vi "serial-read-subVi-safe-copy.vi"() -> ()   [LabVIEW 2021]
uses:
  <vilib>/Instr/_visa.llb/VISA Configure Serial Port (Instr).vi
  SCD41.ctl
  STC31.ctl
  SHT41.ctl
  all-sensor-data.ctl
  SDP810.ctl
panel:
  out "RHT4":T1 {"Humidity (%)" format="%.2f"; "Temp (degC)" format="%.2f"}
  out "RHT3":T1 {"Humidity (%)" format="%.2f"; "Temp (degC)" format="%.2f"}
  out "RHT6":T1 {"Humidity (%)" format="%.2f"; "Temp (degC)" format="%.2f"}
  out "RHT5":T1 {"Humidity (%)" format="%.2f"; "Temp (degC)" format="%.2f"}
  out "CD6":T2 {"CO2 (ppm)" format="%.2f"}
  out "CD5":T2 {"CO2 (ppm)" format="%.2f"}
  out "CD4":T2 {"CO2 (ppm)" format="%.2f"}
  out "CD3":T2 {"CO2 (ppm)" format="%.2f"}
  out "CD2":T3 {"Humidity (%)" format="%.2f"; "Temp (degC)" format="%.2f"; "CO2 (ppm)" format="%.2f"}
  out "CD1":T3 {"Humidity (%)" format="%.2f"; "Temp (degC)" format="%.2f"; "CO2 (ppm)" format="%.2f"}
  out "all-sensor-data":T4 {"dP3"."Temp (degC)" format="%.2f"; "dP3"."dP (mBar)" format="%.2f"; "dP2"."Temp (degC)" format="%.2f"; "dP2"."dP (mBar)" format="%.2f"; "dP1"."Temp (degC)" format="%.2f"; "dP1"."dP (mBar)" format="%.2f"; "CD4"."CO2 (ppm)" format="%.2f"; "CD3"."CO2 (ppm)" format="%.2f"; "RHT4"."Humidity (%)" format="%.2f"; "RHT4"."Temp (degC)" format="%.2f"; "RHT5"."Humidity (%)" format="%.2f"; "RHT5"."Temp (degC)" format="%.2f"; "CD2"."Humidity (%)" format="%.2f"; "CD2"."Temp (degC)" format="%.2f"; "CD2"."CO2 (ppm)" format="%.2f"; "RHT3"."Humidity (%)" format="%.2f"; "RHT3"."Temp (degC)" format="%.2f"; "CD6"."CO2 (ppm)" format="%.2f"; "RHT6"."Humidity (%)" format="%.2f"; "RHT6"."Temp (degC)" format="%.2f"; "CD5"."CO2 (ppm)" format="%.2f"; "CD1"."Humidity (%)" format="%.2f"; "CD1"."Temp (degC)" format="%.2f"; "CD1"."CO2 (ppm)" format="%.2f"}
  in  "state":string
  out "Num Samples":i32
  out "error out":errorcluster
  out "data string array":string[](array[string])
  out "read buffer":string
  out "Bytes Returned":u32
  in  "VISA resource name":refnum<visa-resource-name>="COM22"
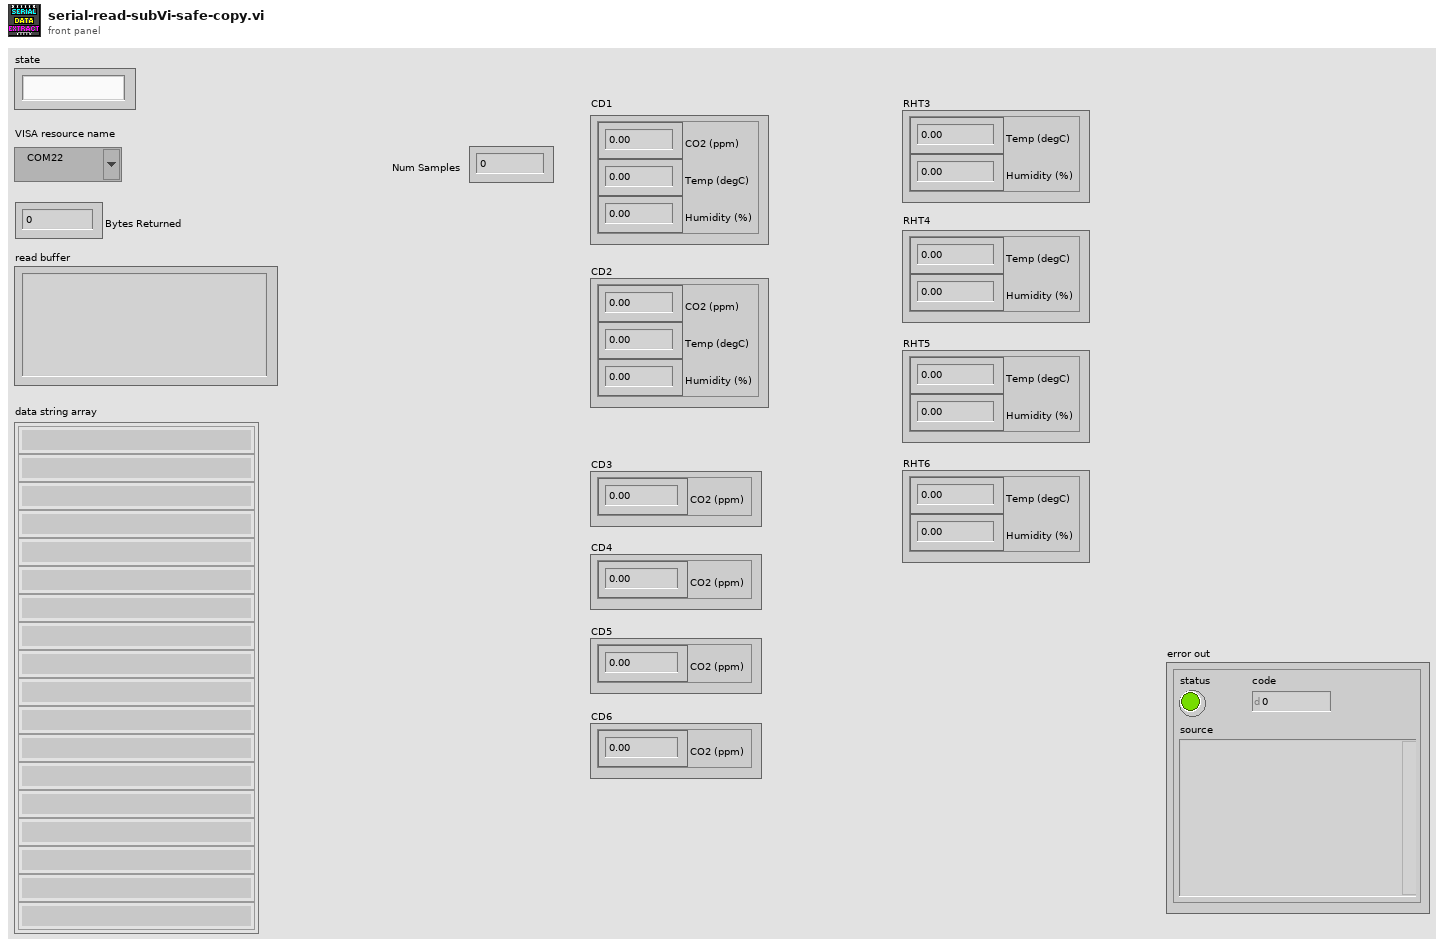
[diagram p1: front panel]
types:
  T1 = typedef "SHT41.ctl" = cluster{"Temp (degC)":dbl, "Humidity (%)":dbl}
  T2 = typedef "STC31.ctl" = cluster{"CO2 (ppm)":dbl}
  T3 = typedef "SCD41.ctl" = cluster{"CO2 (ppm)":dbl, "Temp (degC)":dbl, "Humidity (%)":dbl}
  T4 = typedef "all-sensor-data.ctl" = cluster{"CD1":T3, "CD2":T3, "CD3":T2, "CD4":T2, "CD5":T2, "CD6":T2, "RHT3":T1, "RHT4":T1, "RHT5":T1, "RHT6":T1, "dP1":T5, "dP2":T5, "dP3":T5}
  T5 = typedef "SDP810.ctl" = cluster{"dP (mBar)":dbl, "Temp (degC)":dbl}
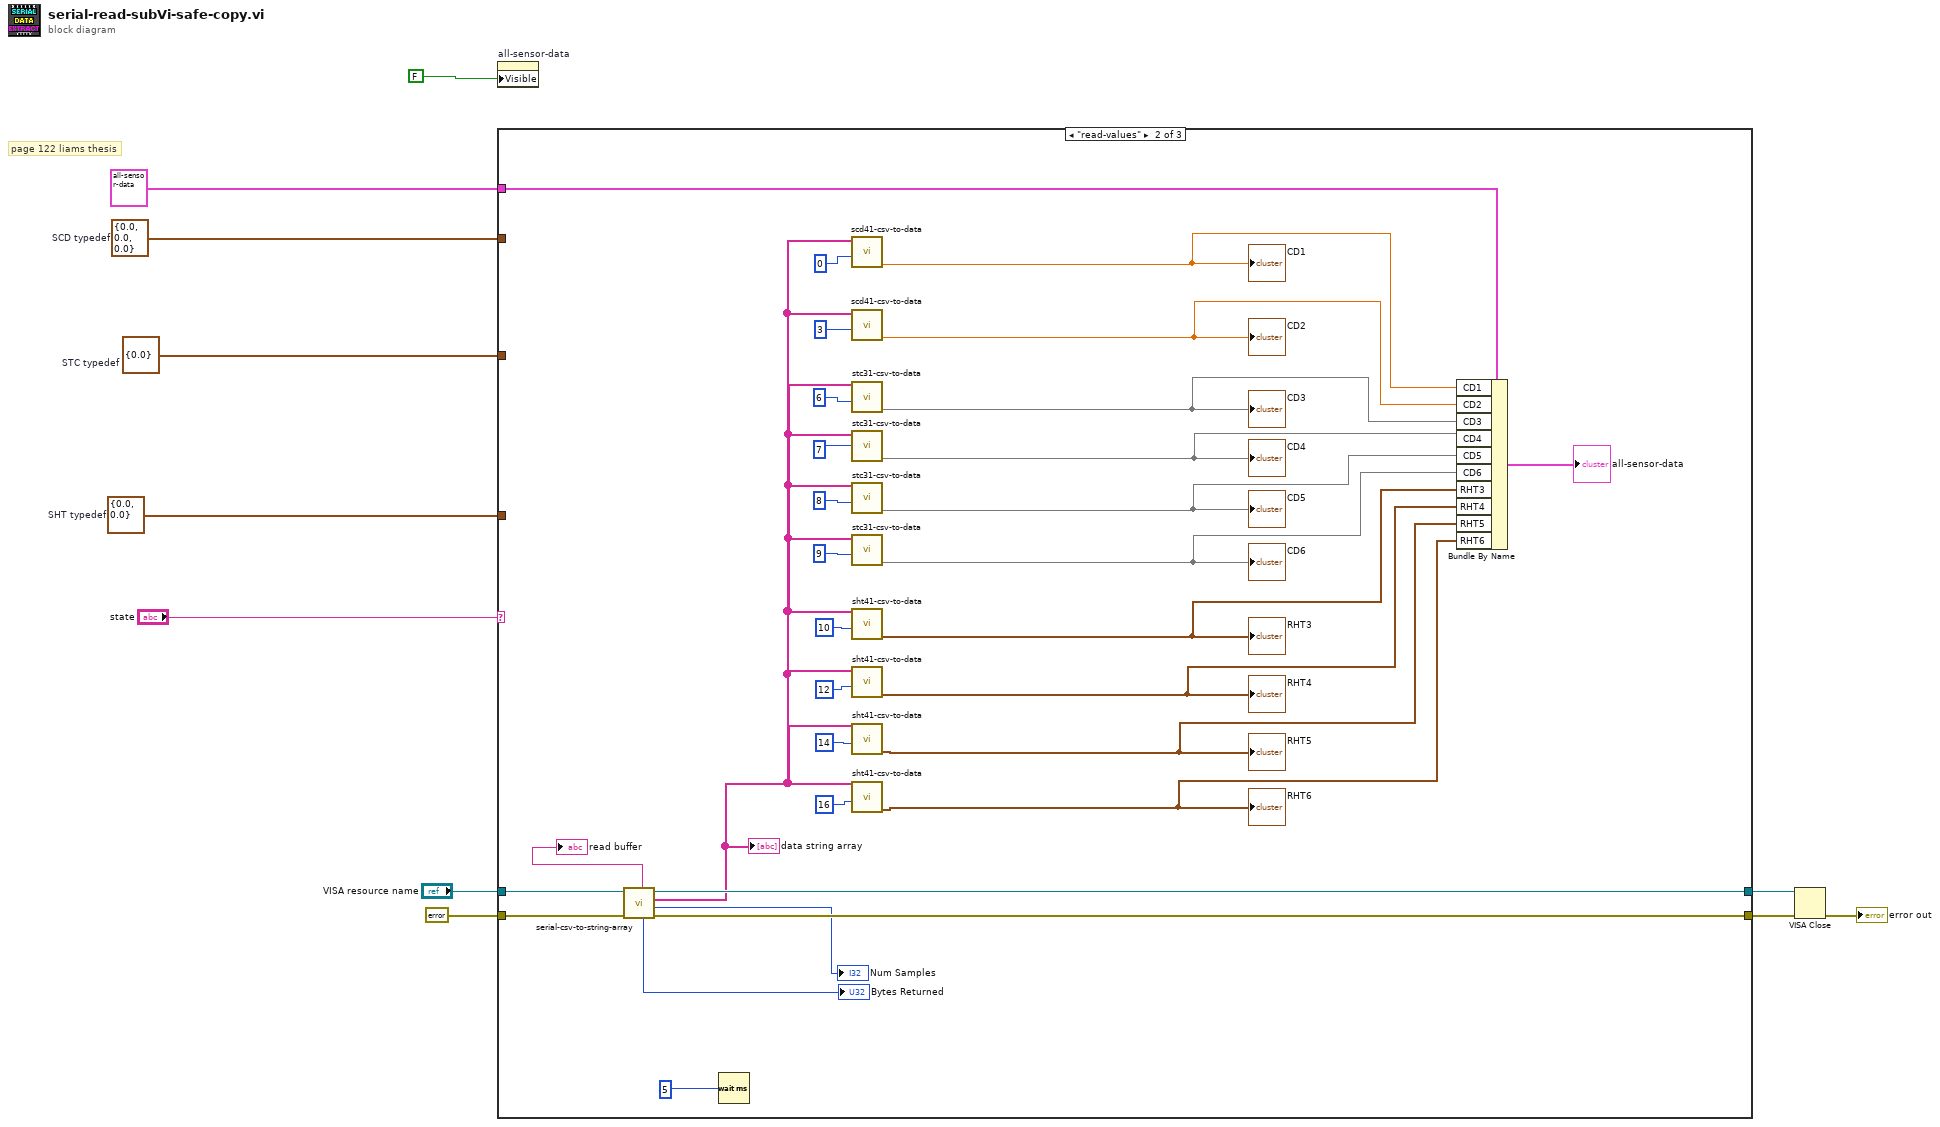
[diagram p0: block diagram]
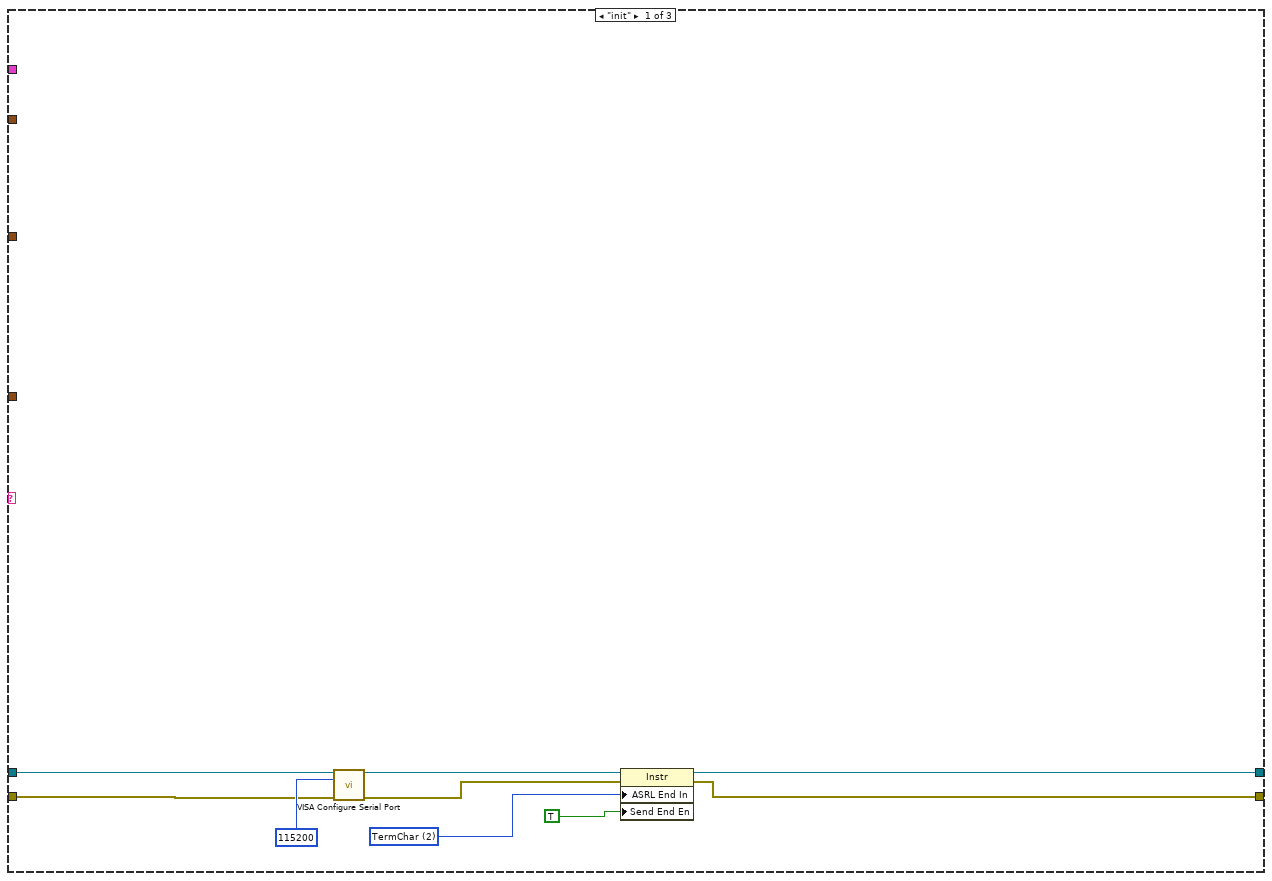
[diagram p2: hidden frame]
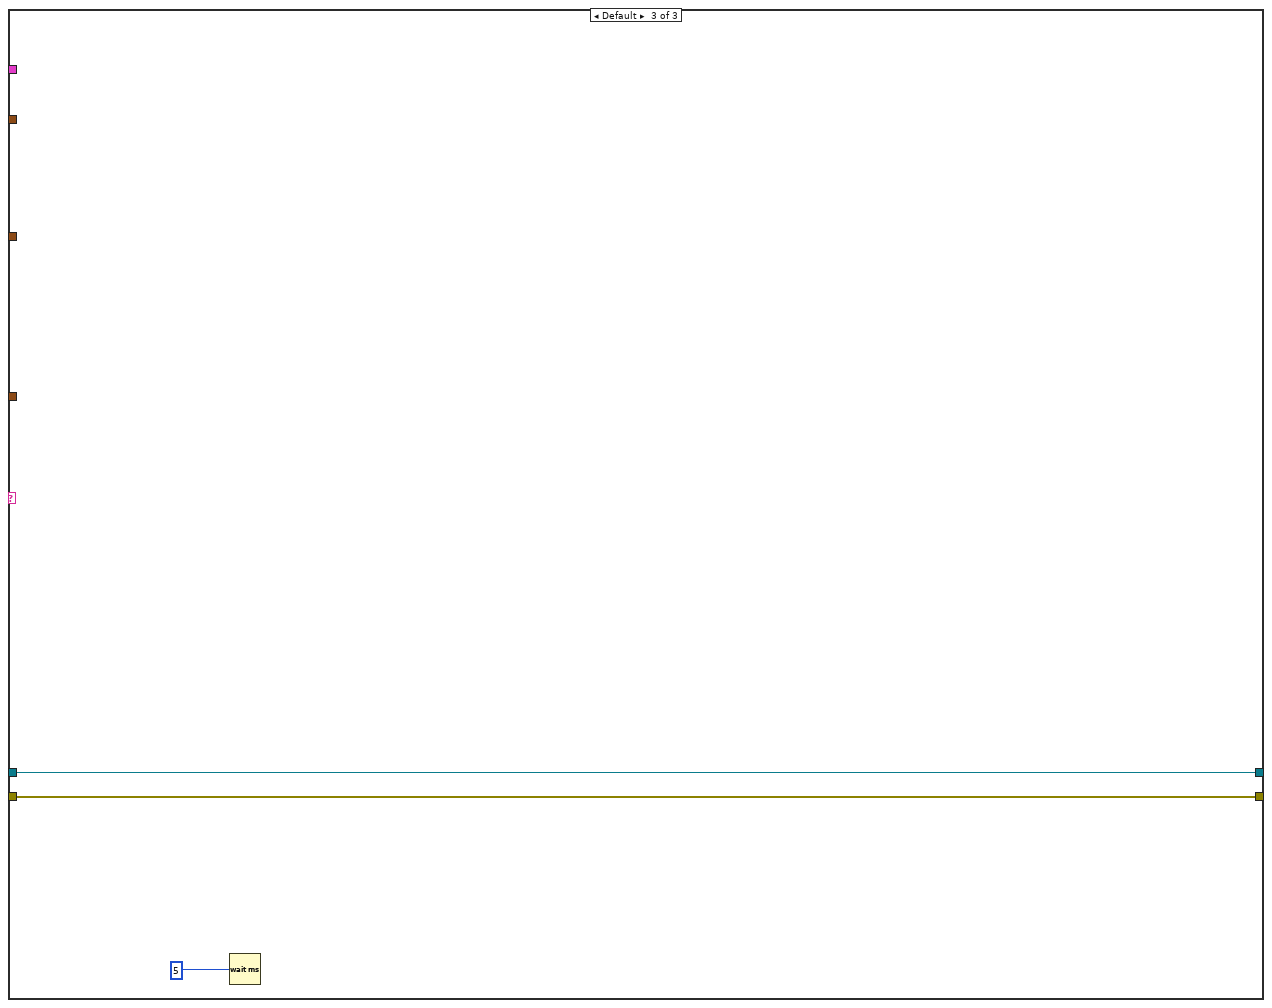
[diagram p3: hidden frame]
diagram:
  w4 = T1 {"Temp (degC)"=0.0, "Humidity (%)"=0.0}  # SHT typedef
  w5 = T2 {"CO2 (ppm)"=0.0}  # STC typedef
  w6 = T3 {"CO2 (ppm)"=0.0, "Temp (degC)"=0.0, "Humidity (%)"=0.0}  # SCD typedef
  # "page 122 liams thesis"
  n1 = property on="all-sensor-data" class="Clust (strict)"("Visible"=FALSE) -> ()  [unwired: 2 in, 2 out]
  n2 = case shown="\"read-values\"" "state" {
    tunnel: [w13 w51 w52] -> w11
    tunnel: [w14 w50 w53] -> w10
    tunnel: "VISA resource name" -> [w15 w36 w53]
    tunnel: w6 -> [_ _ _]
    tunnel: w5 -> [_ _ _]
    tunnel: w4 -> [_ _ _]
    tunnel: T4 {"CD1"={"CO2 (ppm)"=0.0, "Temp (degC)"=0.0, "Humidity (%)"=0.0}, "CD2"={"CO2 (ppm)"=0.0, "Temp (degC)"=0.0, "Humidity (%)"=0.0}, "CD3"={"CO2 (ppm)"=0.0}, "CD4"={"CO2 (ppm)"=0.0}, "CD5"={"CO2 (ppm)"=0.0}, "CD6"={"CO2 (ppm)"=0.0}, "RHT3"={"Temp (degC)"=0.0, "Humidity (%)"=0.0}, "RHT4"={"Temp (degC)"=0.0, "Humidity (%)"=0.0}, "RHT5"={"Temp (degC)"=0.0, "Humidity (%)"=0.0}, "RHT6"={"Temp (degC)"=0.0, "Humidity (%)"=0.0}, "dP1"={"dP (mBar)"=0.0, "Temp (degC)"=0.0}, "dP2"={"dP (mBar)"=0.0, "Temp (degC)"=0.0}, "dP3"={"dP (mBar)"=0.0, "Temp (degC)"=0.0}} ("all-data") -> [_ w38 _]
    tunnel: errorcluster {"status"=FALSE, "code"=0, "source"=""} ("error out") -> [w12 w35 w52]
    frame "init" {
      w18 = u16 2 items=["None", "Last Bit", "TermChar"] ("Serial Settings:End Mode for Reads")
      n3 = call-poly "VISA Configure Serial Port"("VISA resource name"=w15, "baud rate (9600)"=u32 115200, "error in (no error)"=w12) -> ("VISA resource name out"=w19:refnum<visa-resource-name>, "error out"=w20:errorcluster)  [unwired: 11 in]
      n4 = property class="Instr"(reference=w19, error in=w20, "ASRL End In"=w18, "Send End En"=TRUE ("Message Based Settings:Send End Enable")) -> (reference out=w14:refnum<visa-resource-name>, error out=w13:errorcluster)
    }
    frame "read-values" {
      n5 = call "serial-csv-to-string-array.vi"("error in (no error)"=w35, "VISA Refnum in"=w36) -> ("error out"=w51:errorcluster, "timestamp"=→"Num Samples":i32, "data string array"=w34:string[], "VISA Refnum out"=w50:refnum<visa-resource-name>, "Bytes Returned"=→"Bytes Returned":u32, "read buffer"=→"read buffer":string)  [unwired: 4 in]
      "data string array" <- w34
      n6 = Wait (ms)(milliseconds to wait=u32 5) -> ()  [unwired: 1 out]
      n7 = call "scd41-csv-to-data.vi"(9:0 ("Starting Index"), "sensor-csv-input"=w34) -> ("SCD41: Humidity (%)"=w33:dbl)  [unwired: 6 in, 3 out]
      "CD1" <- w33
      n8 = call "scd41-csv-to-data.vi"(9:3 ("Starting Index"), "sensor-csv-input"=w34) -> ("SCD41: Humidity (%)"=w32:dbl)  [unwired: 6 in, 3 out]
      "CD2" <- w32
      n9 = call "stc31-csv-to-data.vi"(9:6 ("index"), "sensor-csv-input"=w34) -> (0:w31)  [unwired: 6 in, 3 out]
      "CD3" <- w31
      n10 = call "stc31-csv-to-data.vi"(9:7 ("Starting Index"), "sensor-csv-input"=w34) -> (0:w30)  [unwired: 6 in, 3 out]
      "CD4" <- w30
      n11 = call "stc31-csv-to-data.vi"(9:8 ("Starting Index"), "sensor-csv-input"=w34) -> (0:w29)  [unwired: 6 in, 3 out]
      "CD5" <- w29
      n12 = call "stc31-csv-to-data.vi"(9:9 ("Starting Index"), "sensor-csv-input"=w34) -> (0:w28)  [unwired: 6 in, 3 out]
      "CD6" <- w28
      n13 = call "sht41-csv-to-data.vi"("Starting Index"=10, "Data In (string array)"=w34) -> ("SHT41: data output"=w27:T1)  [unwired: 7 in, 2 out]
      "RHT3" <- w27
      n14 = call "sht41-csv-to-data.vi"("Starting Index"=12, "Data In (string array)"=w34) -> ("SHT41: data output"=w26:T1)  [unwired: 7 in, 2 out]
      "RHT4" <- w26
      n15 = call "sht41-csv-to-data.vi"("Starting Index"=14, "Data In (string array)"=w34) -> ("SHT41: data output"=w25:T1)  [unwired: 7 in, 2 out]
      "RHT5" <- w25
      n16 = call "sht41-csv-to-data.vi"("Starting Index"=16, "Data In (string array)"=w34) -> ("SHT41: data output"=w24:T1)  [unwired: 7 in, 2 out]
      "RHT6" <- w24
      n17 = Bundle By Name(cluster=w38, "CD1"=w33, "CD2"=w32, "CD3"=w31, "CD4"=w30, "CD5"=w29, "CD6"=w28, "RHT3"=w27, "RHT4"=w26, "RHT5"=w25, "RHT6"=w24) -> (→"all-sensor-data":T4)
    }
    frame Default {
      n18 = Wait (ms)(milliseconds to wait=u32 5) -> ()  [unwired: 1 out]
    }
  }
  n19 = VISA Close(VISA resource name=w10, error in (no error)=w11) -> (error out=→"error out":errorcluster)
